vi "Is Created Queue.vi"(10 "Created Queue Alias":string, 11 "Base Queue in":refnum<class "Base Queue.lvclass">) -> (2 "Is Created Queue?":bool, 3 "Base Queue out":refnum<class "Base Queue.lvclass">)   [LabVIEW 2021, in "jettl.lvlib" / "Base Queue.lvlib" / "Base Queue.lvclass"]
uses:
  Base Queue.lvclass
  C:/git/jettl/src/jettl/jettl/jettl.lvclass
  Base Queue.lvclass/Base Queue.ctl
  Queue Mailbox/Queue Mailbox.lvlib
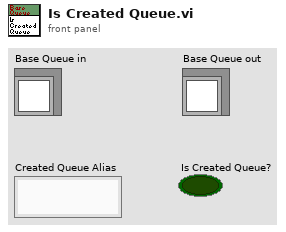
[diagram p1: front panel]
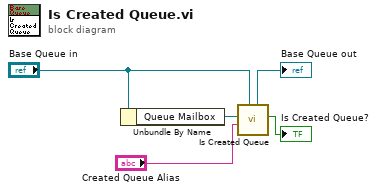
[diagram p0: block diagram]
diagram:
  n1 = Unbundle By Name("Base Queue in") -> ("Queue Mailbox"=w5:refnum<data-value>)
  n2 = call "Is Created Queue.vi"("jettl in"="Base Queue in", "Created Queue Alias"="Created Queue Alias", "Queue Mailbox"=w5) -> ("Is Created Queue?"=→"Is Created Queue?":bool, "jettl out"=→"Base Queue out":refnum<class "Base Queue.lvclass">)  [unwired: 7 in]
